vi "Start Logging.vi"(8 "error in (no error)":errorcluster, 11 "Serial":string) -> (0 "error out":errorcluster)   [LabVIEW 2014]
uses:
  Common/State Machine/State Machine.lvlib
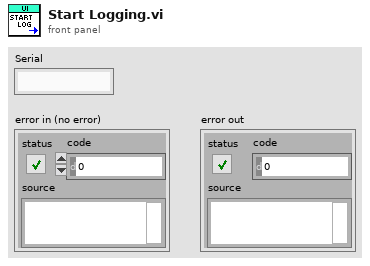
[diagram p1: front panel]
types:
  T1 = cluster{"Serial Number":string, "Test Start":timestamp}
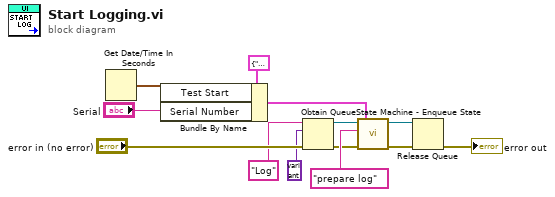
[diagram p0: block diagram]
diagram:
  n1 = Get Date/Time In Seconds() -> (seconds since 1Jan1904=w8:timestamp)
  n2 = Bundle By Name(cluster=T1 {"Serial Number"="", "Test Start"=timestamp(0 s since 1904-01-01)}, "Test Start"=w8, "Serial Number"="Serial") -> (w9:T1)
  n3 = Obtain Queue(name (unnamed)="Log", element data type=variant, error in (no error)="error in (no error)") -> (queue out=w4:refnum<queue>, error out=w3:errorcluster)  [unwired: 2 in, 1 out]
  n4 = call "State Machine - Enqueue State.vi"("error in (no error)"=w3, "Data"=w9, "State"="prepare log", "Queue In"=w4) -> ("error out"=w11:errorcluster, "Queue Out"=w12:refnum<queue>)  [unwired: 6 in]
  n5 = Release Queue(queue=w12, error in (no error)=w11) -> (error out=→"error out":errorcluster)  [unwired: 1 in, 2 out]
